vi "作业1 .vi"() -> ()   [LabVIEW 2017]
uses:
  <vilib>/measure/NI_MABase.lvlib
panel:
  in  "布尔":bool
  out "波形图":waveform(dbl)(graph)
  in  "幅值":dbl(knob) scale=0.0..10.0
  in  "频率":dbl(knob) scale=0.0..10.0
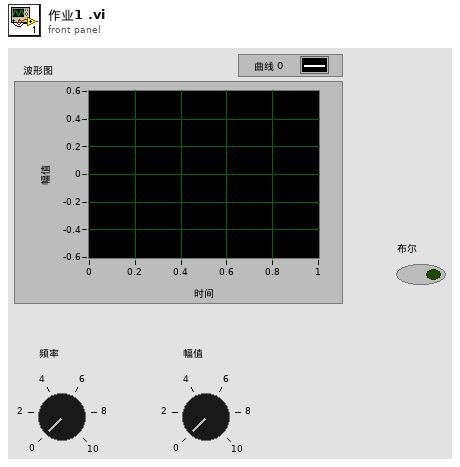
[diagram p1: front panel]
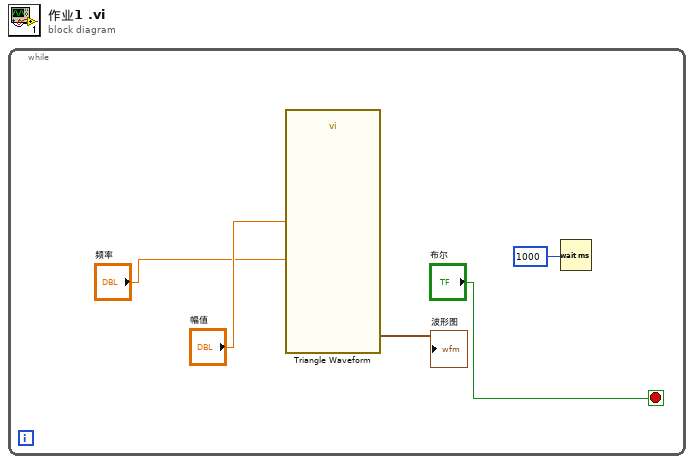
[diagram p0: block diagram]
diagram:
  n1 = while {
    stop <- "布尔" stop-if-true
    n2 = call <vilib>:"Triangle Waveform.vi"("amplitude"="幅值", "frequency"="频率") -> ("signal out"=→"波形图":waveform(dbl))  [unwired: 8 in, 1 out]
    n3 = Wait (ms)(milliseconds to wait=1000) -> ()  [unwired: 1 out]
  }
